vi "GL_ForceBreakPt.vi"(2 "error in":errorcluster, 3 "GL Ref Out":refnum<k7>) -> (0 "error out":errorcluster, 1 "ref out":refnum<k7>)   [LabVIEW 2022 SP3]
uses:
  Command Menu.ctl
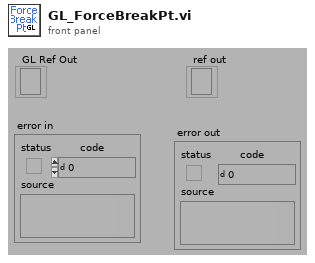
[diagram p1: front panel]
types:
  T1 = typedef "Command Menu.ctl" = enum16{"CommandPassThrough", "Abort Motion", "Define Pos", "Velocity", "Acceleration", "Deceleration", "Position Rel", "Postion Abs", "Begin Move", "After Move", "Home", "KI", "KD", "KP", "IL", "Config I/O", "Set Bit", "Clear Bit", "Motor Off", "Moto On", "Status", "Execute", "Halt Execute", "HX Status", "Tell Velocity", "Check Motion", "BreakPoint", "Tell Position", "Current Code Line", "Tell Switches", "OC Force On", "OC Off", "Pos Soft Limit", "Rev Soft Limit"}
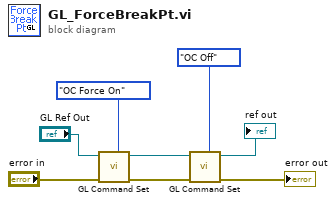
[diagram p0: block diagram]
diagram:
  n1 = call "GL Command Set.vi"("Command"=Command_Menu."OC Force On", "error in (no error)"="error in", "Galil.IGalil"="GL Ref Out") -> ("error out"=w3:errorcluster, "ref out"=w5:refnum<k7>)  [unwired: 4 in, 3 out]
  n2 = call "GL Command Set.vi"("Command"=Command_Menu."OC Off", "error in (no error)"=w3, "Galil.IGalil"=w5) -> ("error out"=→"error out":errorcluster, "ref out"=→"ref out":refnum<k7>)  [unwired: 4 in, 3 out]
